vi "Lock-in auto sensitivity new.vi"(8 "error in (no error)":errorcluster, 9 "milliseconds to wait":u32=1000, 10 "Maximum allowable change":i32=26, 11 "Instrument parameters":T1={"VISA Address"="", "GPIB/TCP Address"="", "String 1"="0_100", "String 2"="0", "Boolean 1"=FALSE, "Boolean 2"=FALSE, "Int 1"=0, "Int 2"=0, "Double 1"=0.0, "Double 2"=0.0}) -> (0 "error out":errorcluster, 2 "Sensitivity out":dbl, 3 "output cluster":T1)   [LabVIEW 2025]
uses:
  TYPE DEFS/S2DS_Instrument parameters.ctl
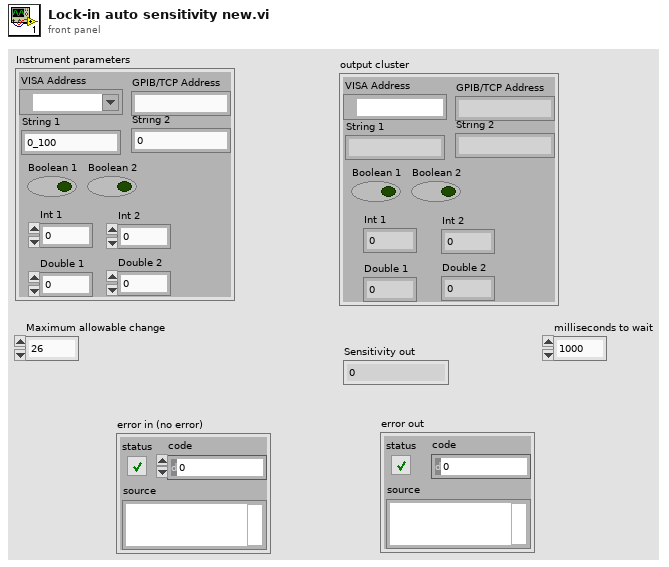
[diagram p1: front panel]
types:
  T1 = typedef "S2DS_Instrument parameters.ctl" = cluster{"VISA Address":refnum<visa-resource-name>, "GPIB/TCP Address":string, "String 1":string, "String 2":string, "Boolean 1":bool, "Boolean 2":bool, "Int 1":i32, "Int 2":i32, "Double 1":dbl, "Double 2":dbl}
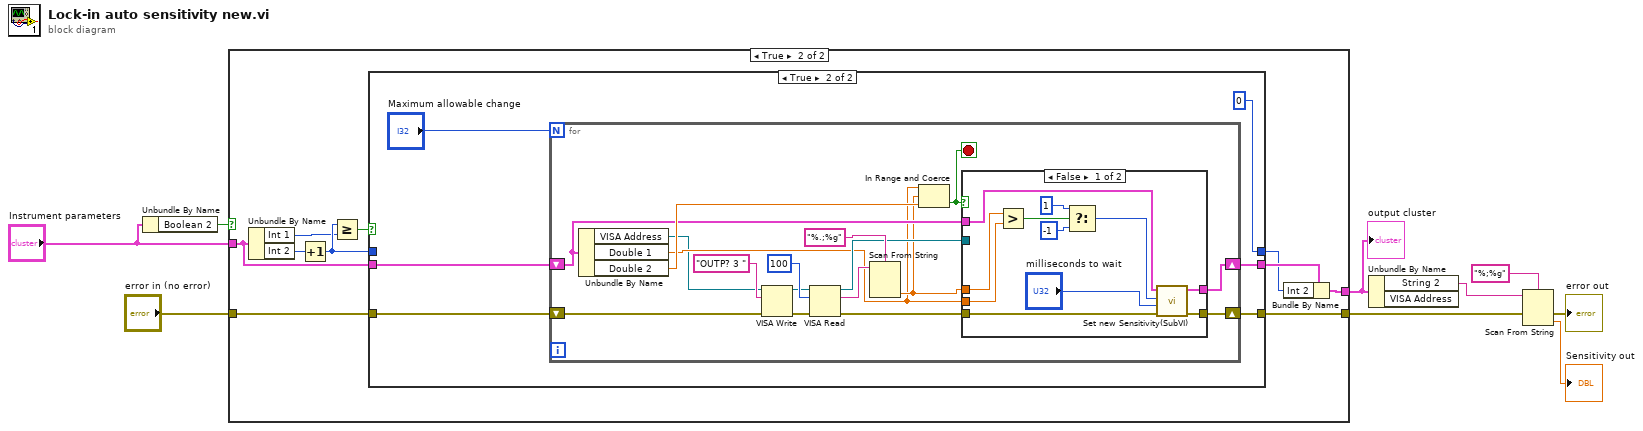
[diagram p0: block diagram]
diagram:
  n1 = Unbundle By Name("Instrument parameters") -> ("Boolean 2"=w9:bool)
  n2 = case shown="True" w9 {
    tunnel: [w10 w21] -> w2
    tunnel: "Instrument parameters" -> [w11 w18]
    tunnel: [w11 w13] -> w6
    tunnel: "error in (no error)" -> [w10 w12]
    frame False {
    }
    frame True {
      n3 = Unbundle By Name(w18) -> ("Int 1"=w17:i32, "Int 2"=w16:i32)
      n4 = Increment(x=w16) -> (x+1=w19:i32)
      n5 = Greater Or Equal?(x=w19, y=w17) -> (x >= y?=w20:bool)
      n6 = case shown="True" w20 {
        tunnel: [w23 w30] -> w21
        tunnel: w12 -> [w23 w26]
        tunnel: [w24 0] -> w14
        tunnel: w19 -> [w24 _]
        tunnel: w18 -> [w22 w28]
        tunnel: [w22 w27] -> w15
        frame False {
        }
        frame True {
          n7 = for {
            N: "Maximum allowable change" -> [_]
            shift-right: [w44] -> w27
            shift-left: w28 -> [w45]
            shift-right: [w47] -> w30
            shift-left: w26 -> [w32]
            stop <- w33 stop-if-true
            n8 = Unbundle By Name(w45) -> ("VISA Address"=w31:refnum<visa-resource-name>, "Double 1"=w34:dbl, "Double 2"=w46:dbl)
            n9 = VISA Write(VISA resource name=w31, write buffer="OUTP? 3 " ("initial string"), error in (no error)=w32) -> (VISA resource name out=w40:refnum<visa-resource-name>, error out=w39:errorcluster)  [unwired: 1 out]
            n10 = VISA Read(VISA resource name=w40, byte count=u32 100, error in (no error)=w39) -> (VISA resource name out=w36:refnum<visa-resource-name>, read buffer=w38:string, error out=w37:errorcluster)  [unwired: 1 out]
            n11 = Scan From String(format string="%.;%g", input string=w38) -> (output 1=w35:dbl)  [unwired: 3 in, 3 out]
            n12 = In Range and Coerce(upper limit=w34, x=w35, lower limit=w46) -> (In Range?=w33:bool)  [unwired: 1 out]
            n13 = case shown="False" w33 {
              tunnel: w36 -> [_ _]
              tunnel: w37 -> [w51 w60]
              tunnel: [w50 w60] -> w47
              tunnel: w45 -> [w52 w59]
              tunnel: [w49 w59] -> w44
              tunnel: w35 -> [w58 _]
              tunnel: w34 -> [w57 _]
              frame False {
                n14 = Greater?(x=w58, y=w57) -> (0:w56:bool)
                n15 = Select(t=1, s=w56, f=-1) -> (s? t:f=w53:i32)
                n16 = call "Set new Sensitivity(SubVI).vi"("error in (no error)"=w51, "milliseconds to wait"="milliseconds to wait", "Numeric"=w53, "Instrument parameters in"=w52) -> ("error out"=w50:errorcluster, "Instrument parameters out"=w49:T1)  [unwired: 5 in, 1 out]
              }
              frame True {
              }
            }
          }
        }
      }
      n17 = Bundle By Name(cluster=w15, "Int 2"=w14) -> (w13:T1)
    }
  }
  "output cluster" <- w6
  n18 = Unbundle By Name(w6) -> ("String 2"=w5:string)  [unwired: 1 out]
  n19 = Scan From String(format string="%;%g", input string=w5, error in=w2) -> (error out=→"error out":errorcluster, output 1=→"Sensitivity out":dbl)  [unwired: 2 in, 2 out]
